vi "Check KFM Connect PLZ.vi"(8 "error in":errorcluster, 11 "Com Port In":T1) -> (0 "error out":errorcluster, 3 "Com Port Out":T1)   [LabVIEW 2018]
uses:
  Data Def/Com Port.ctl
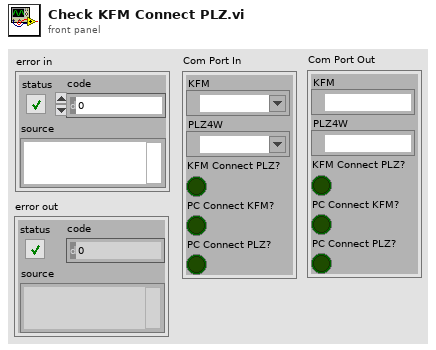
[diagram p1: front panel]
types:
  T1 = typedef "Com Port.ctl" = cluster{"KFM":refnum<visa-resource-name>, "PLZ4W":refnum<visa-resource-name>, "KFM Connect PLZ?":bool, "PC Connect KFM?":bool, "PC Connect PLZ?":bool}
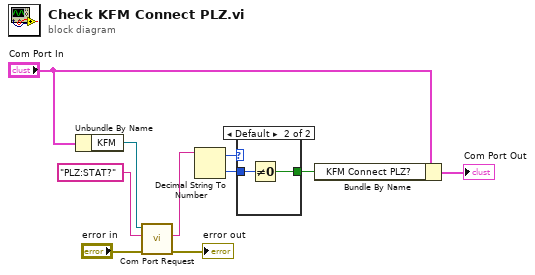
[diagram p0: block diagram]
diagram:
  n1 = Unbundle By Name("Com Port In") -> ("KFM"=w9:refnum<visa-resource-name>)
  n2 = call "Com Port Request.vi"("error in"="error in", "Command"="PLZ:STAT?", "Com Port In"=w9) -> ("error out"=→"error out":errorcluster, "Respond"=w6:string)  [unwired: 6 in, 1 out]
  n3 = Decimal String To Number(string=w6) -> (offset past number=w8:i32, number=w7:i32)  [unwired: 2 in]
  n4 = case shown="Default" w8 {
    tunnel: w7 -> [_ w12]
    tunnel: [_ w11] -> w3
    frame 0 {
    }
    frame Default {
      n5 = Not Equal To 0?(x=w12) -> (x != 0?=w11:bool)
    }
  }
  n6 = Bundle By Name(cluster="Com Port In", "KFM Connect PLZ?"=w3) -> (→"Com Port Out":T1)
